vi "Initialize-NanoDrive-SubVI.vi"() -> (1 "Output Pos Info":T1, 2 "Handle":i32, 3 "ADC/DAC Resolution":u32)   [LabVIEW 2014]
uses:
  lib/Madlib/Madlib.dll
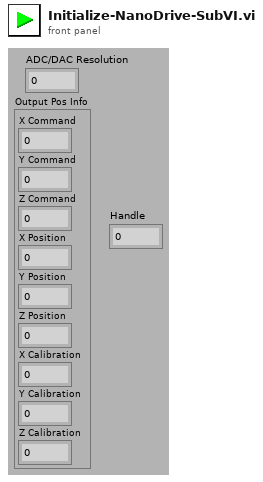
[diagram p1: front panel]
types:
  T1 = cluster{"X Command":dbl, "Y Command":dbl, "Z Command":dbl, "X Position":dbl, "Y Position":dbl, "Z Position":dbl, "X Calibration":dbl, "Y Calibration":dbl, "Z Calibration":dbl}
  T2 = cluster{"position":dbl, "position":dbl, "position":dbl, "position":dbl, "position":dbl, "position":dbl, "Calibration":dbl, "Calibration":dbl, "Calibration":dbl}
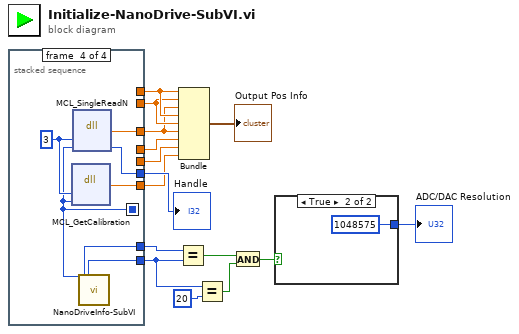
[diagram p0: block diagram]
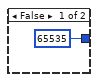
[diagram p2: hidden frame]
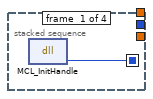
[diagram p3: hidden frame]
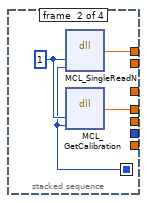
[diagram p4: hidden frame]
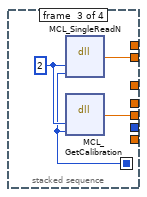
[diagram p5: hidden frame]
diagram:
  n1 = stacked-sequence {
    seq-local: [w16 _ _ _] -> [_ w18 w22 w27]
    tunnel: [_ w20 _ _] -> w4
    tunnel: [_ _ w24 _] -> w3
    tunnel: [_ _ _ w31] -> w2
    tunnel: [_ _ _ w30] -> w15
    tunnel: [_ w17 _ _] -> w14
    tunnel: [_ _ w21 _] -> w13
    tunnel: [_ _ _ w28] -> w12
    tunnel: [_ _ _ w26] -> w11
    tunnel: [_ _ _ w25] -> w10
    frame #0 {
      n2 = dll-call lib="C:/Users/Lambda2/Documents/Softwares/Lambda2/lib/Madlib/Madlib.dll" fn="MCL_InitHandle" label="Madlib.dll:\nMCL_InitHandle"() -> ("handle"=w16:i32)  [unwired: 3 in, 2 out]
    }
    frame #1 {
      w19 = u32 1 ("Axis")
      n3 = dll-call lib="C:/Users/Lambda2/Documents/Softwares/Lambda2/lib/Madlib/Madlib.dll" fn="MCL_SingleReadN"("Axis"=w19, "Handle"=w18) -> ("position"=w20:dbl)  [unwired: 5 in, 2 out]
      n4 = dll-call lib="C:/Users/Lambda2/Documents/Softwares/Lambda2/lib/Madlib/Madlib.dll" fn="MCL_GetCalibration"("Axis"=w19, "Handle"=w18) -> ("Calibration"=w17:dbl)  [unwired: 5 in, 2 out]
    }
    frame #2 {
      w23 = u32 2 ("Axis")
      n5 = dll-call lib="C:/Users/Lambda2/Documents/Softwares/Lambda2/lib/Madlib/Madlib.dll" fn="MCL_SingleReadN"("Axis"=w23, "Handle"=w22) -> ("position"=w24:dbl)  [unwired: 5 in, 2 out]
      n6 = dll-call lib="C:/Users/Lambda2/Documents/Softwares/Lambda2/lib/Madlib/Madlib.dll" fn="MCL_GetCalibration"("Axis"=w23, "Handle"=w22) -> ("Calibration"=w21:dbl)  [unwired: 5 in, 2 out]
    }
    frame #3 {
      w29 = u32 3 ("Axis")
      n7 = dll-call lib="C:/Users/Lambda2/Documents/Softwares/Lambda2/lib/Madlib/Madlib.dll" fn="MCL_GetCalibration"("Axis"=w29, "Handle"=w27) -> ("Calibration"=w28:dbl)  [unwired: 5 in, 2 out]
      n8 = dll-call lib="C:/Users/Lambda2/Documents/Softwares/Lambda2/lib/Madlib/Madlib.dll" fn="MCL_SingleReadN"("Axis"=w29, "Handle"=w27) -> ("position"=w31:dbl, "Handle"=w30:i32)  [unwired: 4 in, 2 out]
      n9 = call "NanoDriveInfo-SubVI.vi"("Handle"=w27) -> ("ADC resolution (bits)"=w26:i16, "DAC resolution (bits)"=w25:i16)  [unwired: 9 in, 16 out]
    }
  }
  "Handle" <- w15
  n10 = Equal?(x=w11, y=w10) -> (x = y?=w8:bool)
  n11 = Bundle("position"=w4, "position"=w3, "position"=w2, "position"=w4, "position"=w3, "position"=w2, "Calibration"=w14, "Calibration"=w13, "Calibration"=w12) -> (→"Output Pos Info":T2)  [unwired: 1 out]
  n12 = Equal?(x=w10, y=i16 20) -> (x = y?=w7:bool)
  n13 = And(x=w8, y=w7) -> (x .and. y?=w6:bool)
  n14 = case shown="True" w6 {
    tunnel: [u16 65535 ("y") u32 1048575 ("y")] -> w5
    frame False {
    }
    frame True {
    }
  }
  "ADC/DAC Resolution" <- w5
